vi "beep150.vi"   [LabVIEW 2010]
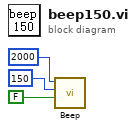
[diagram p0: block diagram]
diagram:
  n1 = call <vilib>:"Beep.vi"("use system alert? (T)"=FALSE, "duration (msec)"=u32 150, "frequency (Hz)"=u32 2000) -> ()  [unwired: 9 in]
